vi "Add Groups.vi"(8 "error in (no error)":errorcluster, 11 "Item Ref in":T1 format="%.0x") -> (0 "error out":errorcluster, 3 "Item Ref out":T1 format="%.0x")   [LabVIEW 2020, in "Modbus Master System Explorer.lvlib"]
uses:
  Modbus Master System Explorer.lvlib
  <vilib>/NI VeriStand/Custom Device API/Custom Device Item Ref.ctl
  Shared/Constants.vi
  <vilib>/NI VeriStand/Custom Device API/Custom Device API.lvlib
  Shared/Modbus Master Shared.lvlib
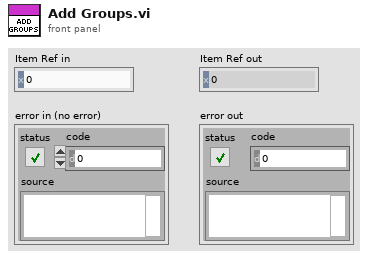
[diagram p1: front panel]
types:
  T1 = typedef "Custom Device API.lvlib/Custom Device Item Ref.ctl" = u64
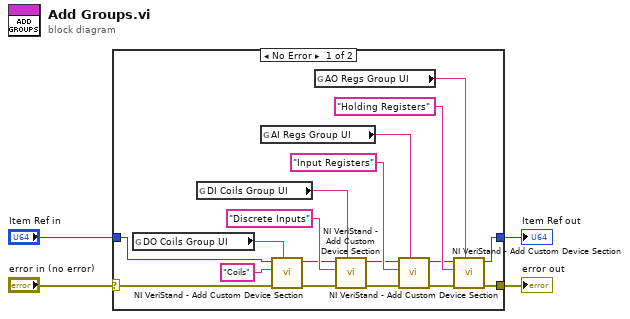
[diagram p0: block diagram]
diagram:
  n1 = case shown="No Error" "error in (no error)" {
    selector: "error in (no error)" -> [w15 w23]
    tunnel: [w9 w24] -> w4
    tunnel: "Item Ref in" -> [w12 w24]
    tunnel: [w10 w23] -> w1
    frame No Error {
      n2 = global read "Constants.vi" "DO Coils Group UI"() -> (w14:string)
      n3 = global read "Constants.vi" "DI Coils Group UI"() -> (w17:string)
      n4 = global read "Constants.vi" "AI Regs Group UI"() -> (w19:string)
      n5 = call <vilib>:"NI VeriStand - Add Custom Device Section.vi"("GUID (Default Section)"=w14, "error in (no error)"=w15, "Section Name"="Coils", "Parent Ref in"=w12) -> ("error out"=w11:errorcluster, "Parent Ref out"=w16:T1)  [unwired: 4 in, 2 out]
      n6 = global read "Constants.vi" "AO Regs Group UI"() -> (w18:string)
      n7 = call <vilib>:"NI VeriStand - Add Custom Device Section.vi"("GUID (Default Section)"=w17, "error in (no error)"=w11, "Section Name"="Discrete Inputs", "Parent Ref in"=w16) -> ("error out"=w8:errorcluster, "Parent Ref out"=w7:T1)  [unwired: 4 in, 2 out]
      n8 = call <vilib>:"NI VeriStand - Add Custom Device Section.vi"("GUID (Default Section)"=w19, "error in (no error)"=w8, "Section Name"="Input Registers", "Parent Ref in"=w7) -> ("error out"=w5:errorcluster, "Parent Ref out"=w6:T1)  [unwired: 4 in, 2 out]
      n9 = call <vilib>:"NI VeriStand - Add Custom Device Section.vi"("GUID (Default Section)"=w18, "error in (no error)"=w5, "Section Name"="Holding Registers", "Parent Ref in"=w6) -> ("error out"=w10:errorcluster, "Parent Ref out"=w9:T1)  [unwired: 4 in, 2 out]
    }
    frame Error {
    }
  }
  "Item Ref out" <- w4
  "error out" <- w1
